vi "ReadDB and update list.vi"(8 "Language":T1, 9 "Currency":T2, 10 "DB Path":path, 11 "MCListbox Refnum":refnum<vi>) -> (1 "Quantity Array":i64[](array[numeric]), 2 "Prices Array":dbl[](array[numeric]), 3 "Names Array":string[](array[string]))   [LabVIEW 2020]
uses:
  Controls/Currency Enum.ctl
  Controls/Language Enum.ctl
  <vilib>/drjdpowell/SQLite Library/SQL Connection/Open (path).vi
  <vilib>/drjdpowell/SQLite Library/SQL Connection/Open (string).vi
  <vilib>/AdvancedString/Path To Command Line String.vi
  <vilib>/drjdpowell/SQLite Library/SQL Connection/Execute SQL (1D DBL results).vi
  <vilib>/drjdpowell/SQLite Library/SQL Connection/Execute SQL (1D String).vi
  <vilib>/drjdpowell/SQLite Library/SQL Connection/Execute SQL (1D Integer results).vi
  <vilib>/drjdpowell/SQLite Library/SQL Connection/Connection.lvclass
  <vilib>/drjdpowell/SQLite Library/SQLite.lvlib
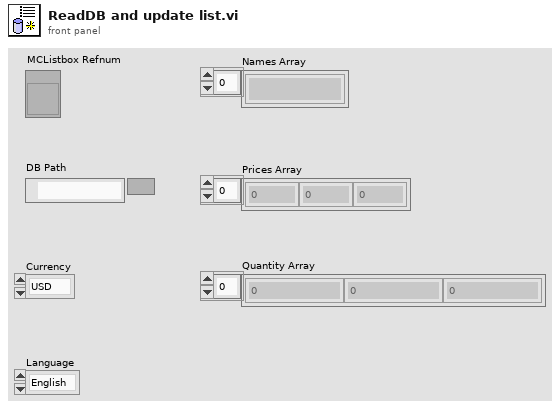
[diagram p1: front panel]
types:
  T1 = typedef "Language Enum.ctl" = enum16{"English", "Español", "Français"}
  T2 = typedef "Currency Enum.ctl" = enum16{"USD", "MXN", "EUR"}
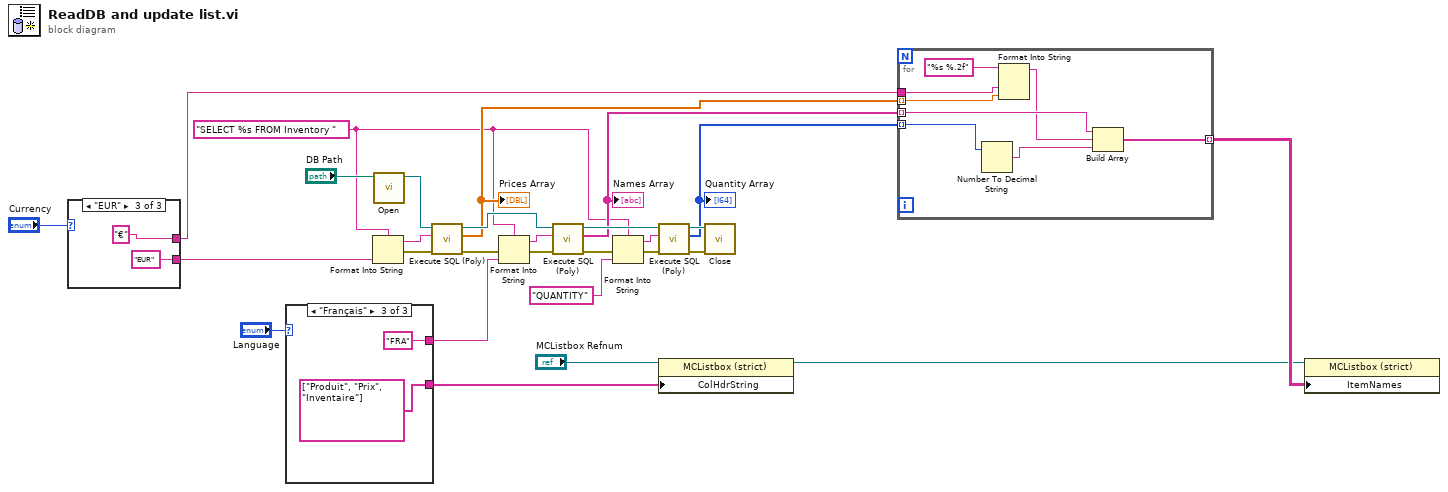
[diagram p0: block diagram]
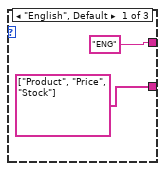
[diagram p2: hidden frame]
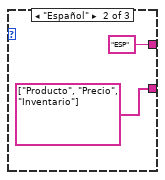
[diagram p3: hidden frame]
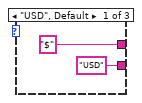
[diagram p4: hidden frame]
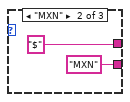
[diagram p5: hidden frame]
diagram:
  w1 = "SELECT %s FROM Inventory " ("format string")
  n1 = case shown="\"EUR\"" "Currency" {
    tunnel: ["USD" "MXN" "EUR"] -> w25
    tunnel: ["$" "$" "€"] -> w4
    frame "USD", Default {
    }
    frame "MXN" {
    }
    frame "EUR" {
    }
  }
  n2 = case shown="\"Français\"" "Language" {
    tunnel: ["ENG" "ESP" "FRA"] -> w20
    tunnel: [string[] ["Product", "Price", "Stock"] ("Column Header Strings[]") string[] ["Producto", "Precio", "Inventario"] ("Column Header Strings[]") string[] ["Produit", "Prix", "Inventaire"] ("Column Header Strings[]")] -> w5
    frame "English", Default {
    }
    frame "Español" {
    }
    frame "Français" {
    }
  }
  n3 = Format Into String(format string=w1, w25) -> (resulting string=w23:string, error out=w14:errorcluster)  [unwired: 2 in]
  n4 = call-poly <vilib>:"Open.vi"("db file"="DB Path") -> ("SQLite Connection"=w24:refnum<class "Connection.lvclass">)  [unwired: 9 in, 1 out]
  n5 = call-poly <vilib>:"Execute SQL (Poly).vi"("error in (no error)"=w14, "SQL"=w23, "SQLite Connection in"=w24) -> ("error out"=w13:errorcluster, "Result Set"=w9:dbl[], "SQLite Connection"=w22:refnum<class "Connection.lvclass">)  [unwired: 5 in, 1 out]
  "Prices Array" <- w9
  n6 = Format Into String(format string=w1, error in=w13, w20) -> (resulting string=w21:string, error out=w12:errorcluster)  [unwired: 1 in]
  n7 = call-poly <vilib>:"Execute SQL (Poly).vi"("error in (no error)"=w12, "SQL"=w21, "SQLite Connection in"=w22) -> ("error out"=w11:errorcluster, "Result Set"=w8:string[], "SQLite Connection"=w19:refnum<class "Connection.lvclass">)  [unwired: 5 in, 1 out]
  "Names Array" <- w8
  n8 = Format Into String(format string=w1, error in=w11, "QUANTITY" ("input 1")) -> (resulting string=w17:string, error out=w10:errorcluster)  [unwired: 1 in]
  n9 = call-poly <vilib>:"Execute SQL (Poly).vi"("error in (no error)"=w10, "SQL"=w17, "SQLite Connection in"=w19) -> ("error out"=w15:errorcluster, "Result Set"=w7:i64[], "SQLite Connection"=w16:refnum<class "Connection.lvclass">)  [unwired: 5 in, 1 out]
  "Quantity Array" <- w7
  n10 = property class="MCListbox (strict)"(reference="MCListbox Refnum", "ColHdrString"=w5) -> (reference out=w2:refnum<vi>)  [unwired: 1 in, 1 out]
  n11 = call-dynamic "Close.vi"("error in (no error)"=w15, "SQLite Connection in"=w16) -> ()  [unwired: 9 in, 1 out]
  n12 = for {
    tunnel: w9 -> [w47] mode=indexing
    tunnel: w8 -> [w45] mode=indexing
    tunnel: w7 -> [w43] mode=indexing
    tunnel: w4 -> [w48]
    tunnel: [w41] -> w3 mode=indexing
    n13 = Number To Decimal String(number=w43) -> (decimal integer string=w42:string)  [unwired: 1 in]
    n14 = Format Into String(format string="%s %.2f", w48, w47) -> (resulting string=w44:string)  [unwired: 2 in, 1 out]
    n15 = Build Array(w45, w44, w42) -> (w41:string[])
  }
  n16 = property class="MCListbox (strict)"(reference=w2, "ItemNames"=w3) -> ()  [unwired: 1 in, 2 out]
